vi "getName.vi"(8 "error in (no error)":errorcluster, 11 "object in":refnum<class "SQLiteConnection.lvclass">) -> (0 "error out":errorcluster, 2 "col name":string, 3 "object out":refnum<class "SQLiteConnection.lvclass">)   [LabVIEW 2019, in "SQLiteConnection.lvclass"]
uses:
  SQLiteConnection.lvclass
  SQLiteConnection.lvclass/SQLiteConnection.ctl
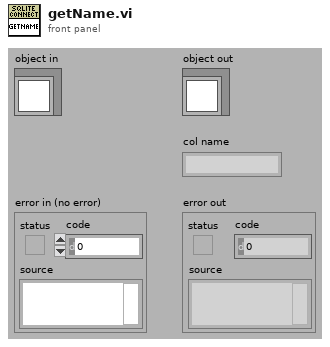
[diagram p1: front panel]
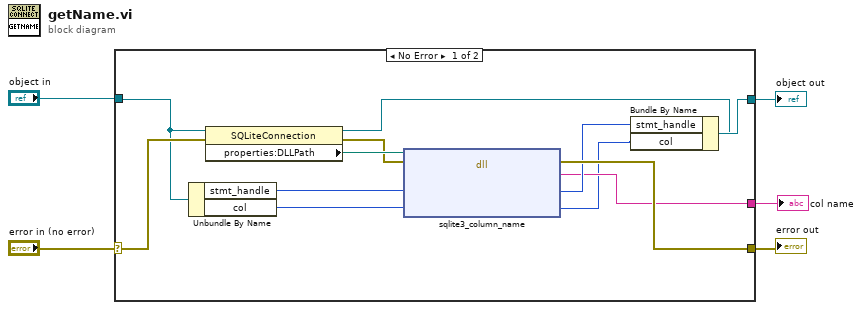
[diagram p0: block diagram]
diagram:
  n1 = case shown="No Error" "error in (no error)" {
    selector: "error in (no error)" -> [w14 w19]
    tunnel: [w9 w19] -> w4
    tunnel: [w17 w18] -> w2
    tunnel: "object in" -> [w11 w18]
    tunnel: [w7 _] -> w1
    frame No Error {
      n2 = Unbundle By Name(w11) -> ("stmt_handle"=w16:u64, "col"=w15:i32)
      n3 = property class="SQLiteConnection"(reference=w11, error in=w14) -> (reference out=w10:refnum<class "SQLiteConnection.lvclass">, error out=w12:errorcluster, "properties:DLLPath"=w13:path)
      n4 = dll-call lib="D:/Users/mcarl/Documents/LabVIEW Projects/OW-PIKO/OW-PIKO Software/sqlite3.dll" fn="sqlite3_column_name"(path in=w13, error in=w12, "stmt_pointer"=w16, "col_int"=w15) -> (error out=w9:errorcluster, "return type"=w7:string, "stmt_pointer"=w8:u64, "col_int"=w6:i32)  [unwired: 1 in, 1 out]
      n5 = Bundle By Name(cluster=w10, "stmt_handle"=w8, "col"=w6) -> (w17:refnum<class "SQLiteConnection.lvclass">)
    }
    frame Error {
    }
  }
  "error out" <- w4
  "object out" <- w2
  "col name" <- w1
